vi "Target.vi"   [LabVIEW 2025]
uses:
  <vilib>/eio/utilities/niEioResolveVilibRelativePath.vi
  <vilib>/rvi/interface/RandomDataEmulation/niFpgaRandomDataHandleErrors.vi
  <vilib>/rvi/Memory/Memory_Emulation/nirvimemoryFastEmulation.vi
  <vilib>/rvi/Memory/Memory_Emulation/nirvimemoryEmulation.vi
  <vilib>/rvi/Emulation/niFpgaEmulationIsFPGAContextNoSignature.vi
  <vilib>/rvi/DataTransferAndStorage/Container/Common/niFpgaContainerGetUniqueNameForEmu.vi
  <vilib>/rvi/Emulation/niFpgaProcessEmulError.vi
  <vilib>/rvi/Emulation/niFpgaSctlEmulationGetInTimedLoop.vi
  <vilib>/rvi/errors/nirviReportUnexpectedCaseInternalError (U32).vi
  <vilib>/rvi/DataTransferAndStorage/Container/XNode/niFpgaContainer.xnode
  <vilib>/rvi/interface/RandomDataEmulation/nirviRandomDataFpgaReadWriteTemplate.vi
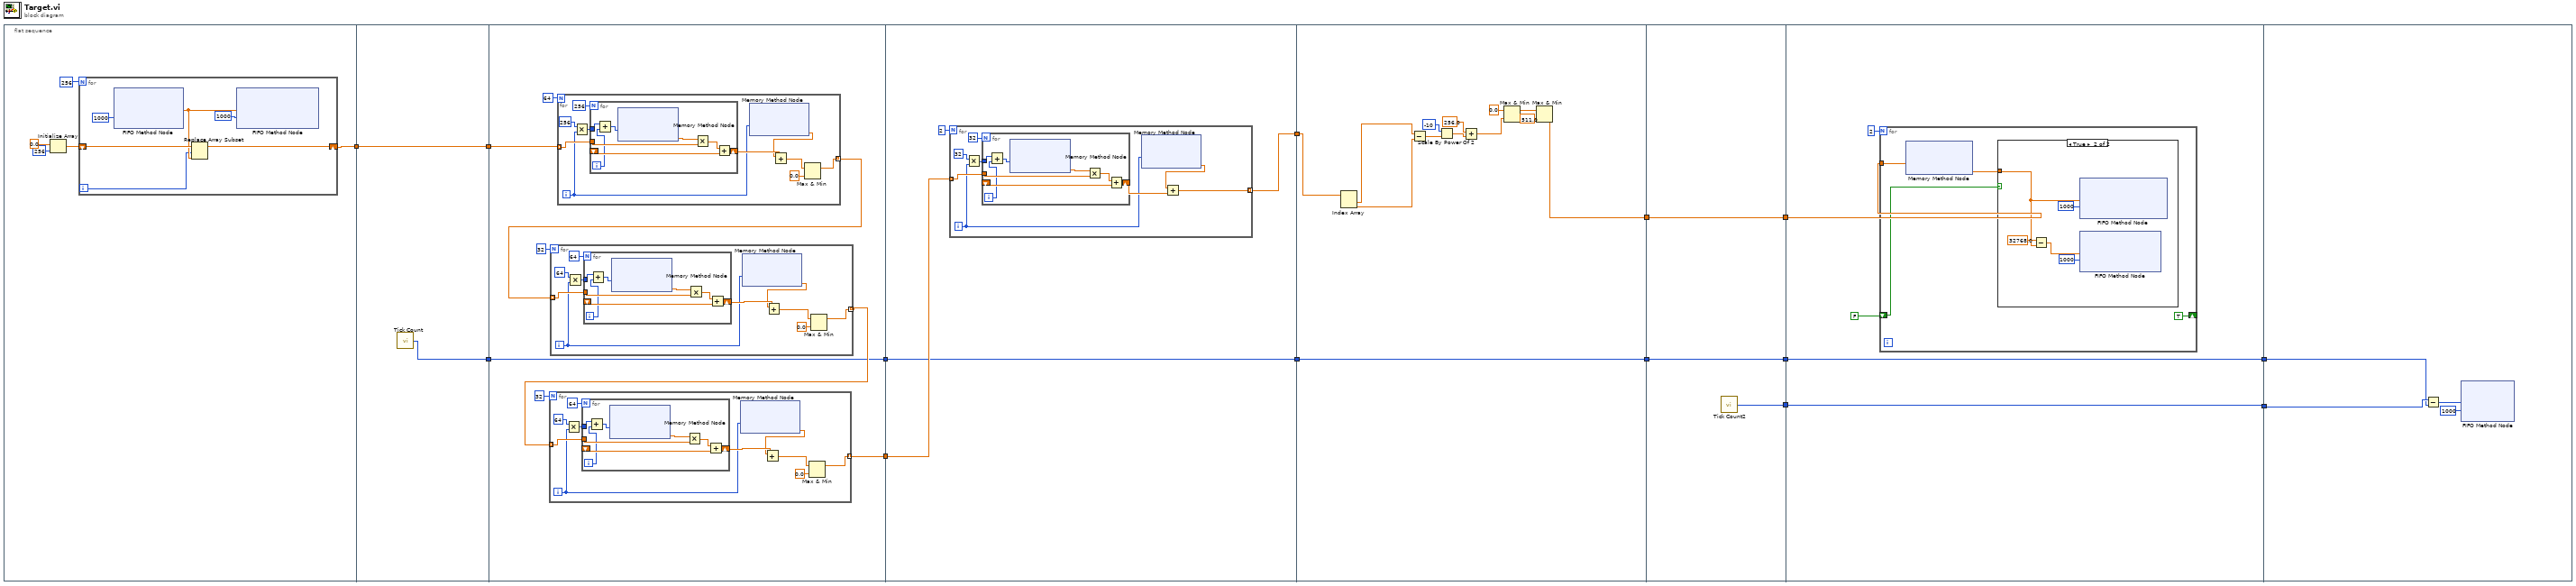
[diagram p0: block diagram]
diagram:
  n1 = flat-sequence {
    tunnel: [w18] -> w8
    tunnel: w8 -> [w27]
    tunnel: [w27] -> w7
    tunnel: [w26] -> w6
    tunnel: w7 -> [w30]
    tunnel: [w29] -> w14
    tunnel: w6 -> [w28]
    tunnel: [w28] -> w11
    tunnel: w14 -> [w92]
    tunnel: [w91] -> w13
    tunnel: w11 -> [w90]
    tunnel: [w90] -> w10
    tunnel: w13 -> [w112]
    tunnel: [w111] -> w5
    tunnel: w10 -> [w110]
    tunnel: [w110] -> w3
    tunnel: w5 -> [w125]
    tunnel: [w125] -> w4
    tunnel: w3 -> [w124]
    tunnel: [w124] -> w2
    tunnel: [w123] -> w1
    tunnel: w4 -> [w129]
    tunnel: [w126] -> w12
    tunnel: w2 -> [w127]
    tunnel: [w127] -> w9
    tunnel: w1 -> [w126]
    tunnel: w12 -> [w143]
    tunnel: w9 -> [w142]
    frame #0 {
      n2 = Initialize Array(sgl 0.0 ("element"), 256 ("dimension size")) -> (w15:sgl[])
      n3 = for {
        N: 256 -> [_]
        shift-right: [w21] -> w18
        shift-left: w15 -> [w23]
        i -> [w20]
        n4 = xnode ("FIFO Method Node")("Timeout"=1000) -> ("Element"=w22:sgl)  [unwired: 1 in, 2 out]
        n5 = Replace Array Subset(array=w23, new element=w22, index=w20) -> (w21:sgl[])
        n6 = xnode ("FIFO Method Node")("Element"=w22, "Timeout"=1000) -> ()  [unwired: 1 in, 2 out]
      }
    }
    frame #1 {
      n7 = call "Tick Count"() -> ("Tick Count(uSec)"=w26:u32)
    }
    frame #2 {
      n8 = for {
        N: 64 -> [_]
        tunnel: w30 -> [w81] mode=indexing
        tunnel: [w72] -> w34 mode=indexing
        i -> [w76]
        n9 = Multiply(x=256, y=w76) -> (x*y=w75:i32)
        n10 = for {
          N: 256 -> [_]
          tunnel: w81 -> [w87]
          shift-right: [w86] -> w79
          shift-left: _ -> [w85]
          tunnel: w75 -> [w84]
          i -> [w83]
          n11 = Add(x=w84, y=w83) -> (x+y=w82:i32)
          n12 = xnode ("Memory Method Node")("Address"=w82) -> ("Data"=w89:sgl)  [unwired: 1 in, 1 out]
          n13 = Multiply(x=w89, y=w87) -> (x*y=w88:sgl)
          n14 = Add(x=w88, y=w85) -> (x+y=w86:sgl)
        }
        n15 = xnode ("Memory Method Node")("Address"=w76) -> ("Data"=w78:sgl)  [unwired: 1 in, 1 out]
        n16 = Add(x=w78, y=w79) -> (x+y=w74:sgl)
        n17 = Max & Min(x=w74, y=sgl 0.0) -> (max(x,y)=w72:sgl)  [unwired: 1 out]
      }
      n18 = for {
        N: 32 -> [_]
        tunnel: w34 -> [w63] mode=indexing
        tunnel: [w54] -> w35 mode=indexing
        i -> [w58]
        n19 = Multiply(x=64, y=w58) -> (x*y=w57:i32)
        n20 = for {
          N: 64 -> [_]
          tunnel: w63 -> [w69]
          shift-right: [w68] -> w61
          shift-left: _ -> [w67]
          tunnel: w57 -> [w66]
          i -> [w65]
          n21 = Add(x=w66, y=w65) -> (x+y=w64:i32)
          n22 = xnode ("Memory Method Node")("Address"=w64) -> ("Data"=w71:sgl)  [unwired: 1 in, 1 out]
          n23 = Multiply(x=w71, y=w69) -> (x*y=w70:sgl)
          n24 = Add(x=w70, y=w67) -> (x+y=w68:sgl)
        }
        n25 = xnode ("Memory Method Node")("Address"=w58) -> ("Data"=w60:sgl)  [unwired: 1 in, 1 out]
        n26 = Add(x=w60, y=w61) -> (x+y=w55:sgl)
        n27 = Max & Min(x=w55, y=sgl 0.0) -> (max(x,y)=w54:sgl)  [unwired: 1 out]
      }
      n28 = for {
        N: 32 -> [_]
        tunnel: w35 -> [w45] mode=indexing
        tunnel: [w36] -> w29 mode=indexing
        i -> [w40]
        n29 = Multiply(x=64, y=w40) -> (x*y=w39:i32)
        n30 = for {
          N: 64 -> [_]
          tunnel: w45 -> [w51]
          shift-right: [w50] -> w43
          shift-left: _ -> [w49]
          tunnel: w39 -> [w48]
          i -> [w47]
          n31 = Add(x=w48, y=w47) -> (x+y=w46:i32)
          n32 = xnode ("Memory Method Node")("Address"=w46) -> ("Data"=w53:sgl)  [unwired: 1 in, 1 out]
          n33 = Multiply(x=w53, y=w51) -> (x*y=w52:sgl)
          n34 = Add(x=w52, y=w49) -> (x+y=w50:sgl)
        }
        n35 = xnode ("Memory Method Node")("Address"=w40) -> ("Data"=w42:sgl)  [unwired: 1 in, 1 out]
        n36 = Add(x=w42, y=w43) -> (x+y=w37:sgl)
        n37 = Max & Min(x=w37, y=sgl 0.0) -> (max(x,y)=w36:sgl)  [unwired: 1 out]
      }
    }
    frame #3 {
      n38 = for {
        N: 2 -> [_]
        tunnel: w92 -> [w101] mode=indexing
        tunnel: [w94] -> w91 mode=indexing
        i -> [w96]
        n39 = Multiply(x=32, y=w96) -> (x*y=w95:i32)
        n40 = for {
          N: 32 -> [_]
          tunnel: w101 -> [w107]
          shift-right: [w106] -> w99
          shift-left: _ -> [w105]
          tunnel: w95 -> [w104]
          i -> [w103]
          n41 = Add(x=w104, y=w103) -> (x+y=w102:i32)
          n42 = xnode ("Memory Method Node")("Address"=w102) -> ("Data"=w109:sgl)  [unwired: 1 in, 1 out]
          n43 = Multiply(x=w109, y=w107) -> (x*y=w108:sgl)
          n44 = Add(x=w108, y=w105) -> (x+y=w106:sgl)
        }
        n45 = xnode ("Memory Method Node")("Address"=w96) -> ("Data"=w98:sgl)  [unwired: 1 in, 1 out]
        n46 = Add(x=w98, y=w99) -> (x+y=w94:sgl)
      }
    }
    frame #4 {
      n47 = Index Array(array=w112) -> (element #1=w117:sgl, element #2=w118:sgl)  [unwired: 2 in]
      n48 = Subtract(x=w117, y=w118) -> (x-y=w119:sgl)
      n49 = Scale By Power Of 2(n=i16 -10, x=w119) -> (x*2^n=w120:sgl)
      n50 = Add(x=sgl 256.0, y=w120) -> (x+y=w121:sgl)
      n51 = Max & Min(x=sgl 0.0, y=w121) -> (max(x,y)=w122:sgl)  [unwired: 1 out]
      n52 = Max & Min(x=w122, y=sgl 511.0) -> (min(x,y)=w111:sgl)  [unwired: 1 out]
    }
    frame #5 {
      n53 = call "Tick Count2"() -> ("Tick Count(uSec)"=w123:u32)
    }
    frame #6 {
      n54 = for {
        N: 2 -> [_]
        tunnel: w129 -> [w134]
        shift-right: [TRUE] -> _
        shift-left: FALSE -> [w133]
        n55 = xnode ("Memory Method Node")("Address"=w134) -> ("Data"=w131:sgl)  [unwired: 1 in, 1 out]
        n56 = case shown="True" w133 {
          tunnel: w131 -> [_ w135]
          frame False {
          }
          frame True {
            n57 = Subtract(x=sgl 32768.0, y=w135) -> (x-y=w139:sgl)
            n58 = xnode ("FIFO Method Node")("Element"=w135, "Timeout"=1000) -> ()  [unwired: 1 in, 2 out]
            n59 = xnode ("FIFO Method Node")("Element"=w139, "Timeout"=1000) -> ()  [unwired: 1 in, 2 out]
          }
        }
      }
    }
    frame #7 {
      n60 = Subtract(x=w143, y=w142) -> (x-y=w141:u32)
      n61 = xnode ("FIFO Method Node")("Element"=w141, "Timeout"=1000) -> ()  [unwired: 1 in, 2 out]
    }
  }
